vi "DifferentialPositionDutyCycle SetControl.vi"(0 "DeviceReference":T1, 1 "TargetPosition":dbl, 2 "DifferentialPosition":dbl, 3 "EnableFOC":bool=TRUE, 4 "TargetSlot":i32, 5 "DifferentialSlot":i32=1, 6 "OverrideBrakeDurNeutral":bool, 7 "error in":errorcluster, 8 "LimitForwardMotion":bool, 9 "LimitReverseMotion":bool, 10 "IgnoreHardwareLimits":bool, 11 "UseTimesync":bool, 18 "Update Frequency (Hz)":dbl=100.0) -> (20 "DeviceReference Out":T1, 27 "error out":errorcluster)   [LabVIEW 2023]
doc: "Request PID to target position with a differential position setpoint.\nThis control mode will set the motor's position setpoint to the position specified by the user. It will also set the motor's differential position setpoint to the specified position."
uses:
  <vilib>/Rock Robotics/WPI/ThirdParty/Phoenix6/DeviceReference.ctl
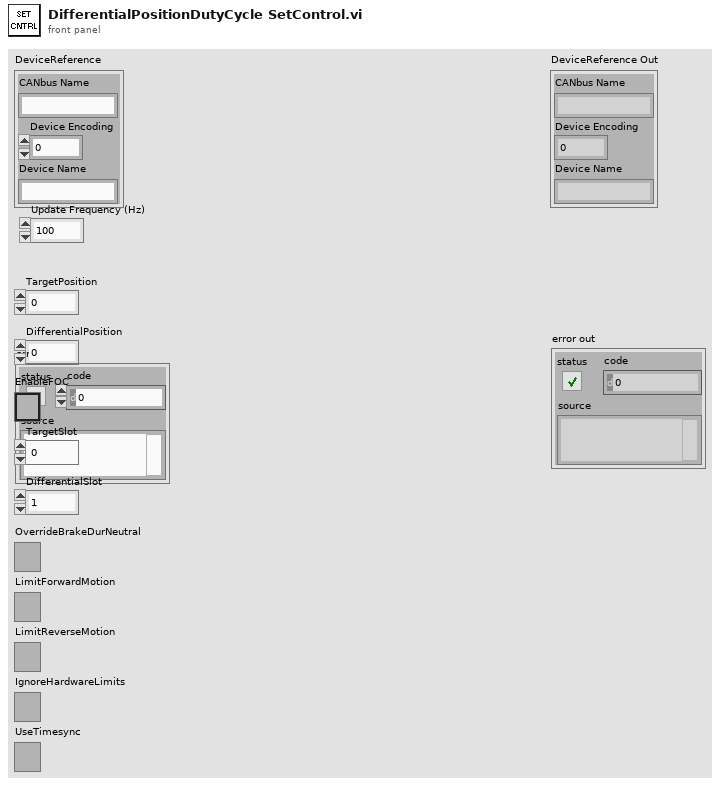
[diagram p1: front panel]
types:
  T1 = typedef "DeviceReference.ctl" = cluster{"CANbus Name":string, "Device Encoding":u32, "Device Name":string}
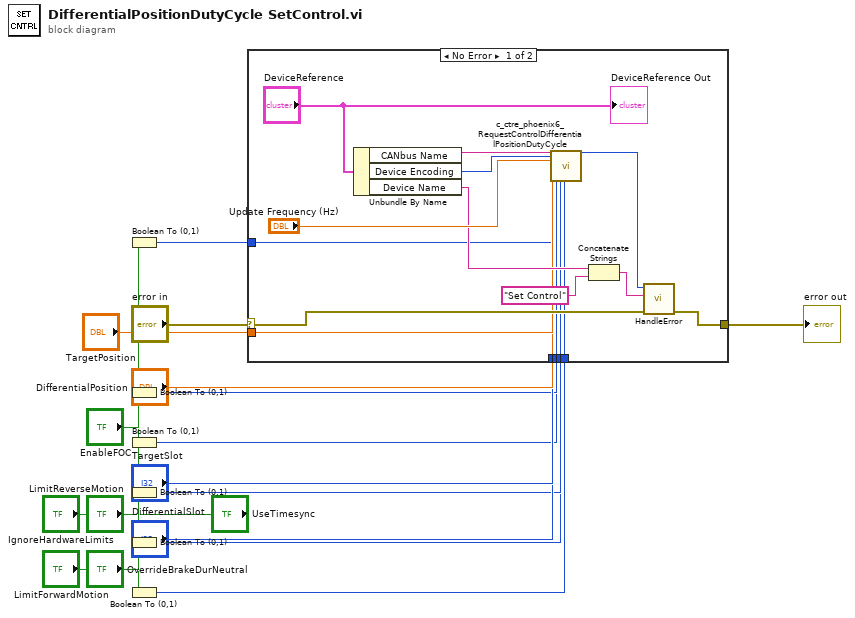
[diagram p0: block diagram]
diagram:
  n1 = Boolean To (0,1)(Boolean="EnableFOC") -> (0, 1=w13:i16)
  n2 = Boolean To (0,1)(Boolean="OverrideBrakeDurNeutral") -> (0, 1=w9:i16)
  n3 = Boolean To (0,1)(Boolean="LimitForwardMotion") -> (0, 1=w7:i16)
  n4 = Boolean To (0,1)(Boolean="LimitReverseMotion") -> (0, 1=w5:i16)
  n5 = Boolean To (0,1)(Boolean="IgnoreHardwareLimits") -> (0, 1=w3:i16)
  n6 = Boolean To (0,1)(Boolean="UseTimesync") -> (0, 1=w1:i16)
  n7 = case shown="No Error" "error in" {
    selector: "error in" -> [w33 w39]
    tunnel: [w32 w39] -> w17
    tunnel: "TargetPosition" -> [w28 _]
    tunnel: "DifferentialPosition" -> [w27 _]
    tunnel: w13 -> [w26 _]
    tunnel: "TargetSlot" -> [w25 _]
    tunnel: "DifferentialSlot" -> [w24 _]
    tunnel: w9 -> [w23 _]
    tunnel: w7 -> [w22 _]
    tunnel: w5 -> [w21 _]
    tunnel: w3 -> [w20 _]
    tunnel: w1 -> [w19 _]
    frame No Error {
      n8 = Unbundle By Name("DeviceReference") -> ("CANbus Name"=w37:string, "Device Encoding"=w36:u32, "Device Name"=w31:string)
      n9 = call <vilib>:"c_ctre_phoenix6_RequestControlDifferentialPositionDutyCycle.vi"("String 2"=w37, "Numeric 2"=w36, "Numeric 3"="Update Frequency (Hz)", "Numeric 4"=w28, "Numeric 5"=w27, "Numeric 6"=w26, "Numeric 7"=w25, "Numeric 8"=w24, "Numeric 9"=w23, "Numeric 10"=w22, "Numeric 11"=w21, "Numeric 12"=w20, "Numeric 13"=w19) -> ("Numeric"=w34:i32)  [unwired: 13 in, 1 out]
      n10 = Concatenate Strings(w31, "Set Control" ("origin")) -> (w29:string)
      n11 = call <vilib>:"HandleError.vi"("error in"=w33, "origin"=w29, "Status"=w34) -> ("error out"=w32:errorcluster)  [unwired: 8 in]
      "DeviceReference Out" <- "DeviceReference"
    }
    frame Error {
    }
  }
  "error out" <- w17
